vi "Test Executives to Data Type.vi"(8 "error in (no error)":errorcluster, 11 "Test Executive Refs":refnum<data-value>[](array[refnum])) -> (0 "error out":errorcluster, 3 "Boolean out":refnum<class "Test Executive 1D.lvclass">)   [LabVIEW 2017, in "Custom Type Test Executive.lvlib" / "Test Executive 1D.lvclass"]
uses:
  <vilib>/gpm_packages/@cs/test-executive/Source/Custom Type Test Executive/Test Executive 1D Data Type/Test Executive 1D.lvclass
  <vilib>/gpm_packages/@cs/test-executive/Source/Test Executive/ITestExecutive/ITest Executive.lvclass
  <vilib>/gpm_packages/@cs/test-executive/Source/Custom Type Test Executive/Test Executive 1D Data Type/Test Executive 1D.lvclass/Test Executive 1D.ctl
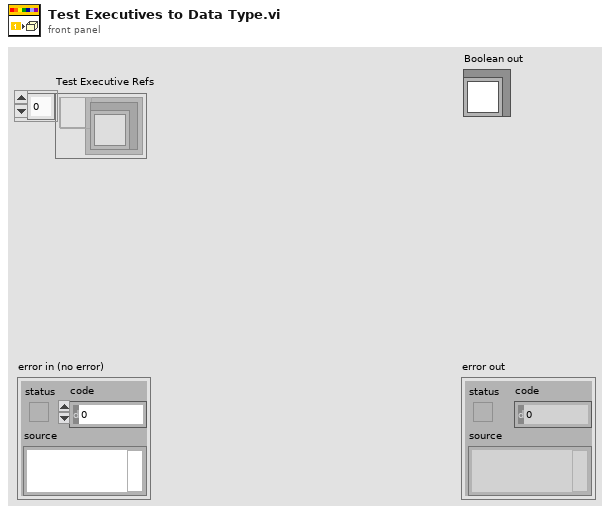
[diagram p1: front panel]
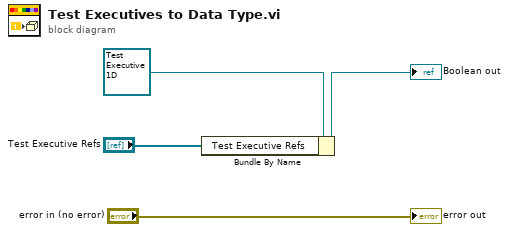
[diagram p0: block diagram]
diagram:
  n1 = Bundle By Name(cluster=refnum<class "Test Executive 1D.lvclass"> refnum ("Boolean in"), "Test Executive Refs"="Test Executive Refs") -> (→"Boolean out":refnum<class "Test Executive 1D.lvclass">)
  "error out" <- "error in (no error)"
